vi "Initialize.vi"(7 "ChannelName":string="Setpoint.ch%d.SP", 8 "error in":errorcluster, 9 "Number of Channels":u32=1, 10 "Instance Name":string, 11 "Chiller in":refnum<class "Chiller.lvclass">) -> (0 "error out":errorcluster, 2 "Channel":T1[](array[typedef]), 3 "Chiller out":refnum<class "Chiller.lvclass">)   [LabVIEW 2023, in "Chiller.lvclass"]
uses:
  Chiller.lvclass
  Utilities/Channel.ctl
  Chiller.lvclass/Chiller.ctl
  Low Level Capabilities/OnOff/OnOff.lvclass
  Low Level Capabilities/Error/Error.lvclass
  Low Level Capabilities/Error Channels/Error Channels.lvclass
  Low Level Capabilities/Temperature/Temperature Actual Value/Temperature Actual Value.lvclass
  Low Level Capabilities/Temperature/Temperature Gradient/Temperature Gradient.lvclass
  Low Level Capabilities/Temperature/Temperature Limit/Temperature Limit.lvclass
  Low Level Capabilities/Temperature/Temperature Setpoint/Temperature Setpoint.lvclass
  Low Level Capabilities/Pressure/Pressure Actual Value/Pressure Actual Value.lvclass
  Low Level Capabilities/Pressure/Pressure Gradient/Pressure Gradient.lvclass
  Low Level Capabilities/Pressure/Pressure Limit/Pressure Limit.lvclass
  Low Level Capabilities/Pressure/Pressure Setpoint/Pressure Setpoint.lvclass
  Low Level Capabilities/Flow/Flow Actual Value/Flow Actual Value.lvclass
  Low Level Capabilities/Flow/Flow Gradient/Flow Gradient.lvclass
  Low Level Capabilities/Flow/Flow Limit/Flow Limit.lvclass
  Low Level Capabilities/Flow/Flow Setpoint/Flow Setpoint.lvclass
  Low Level Capabilities/Control Mode/Control Mode.lvclass
  Low Level Capabilities/Output Enable/Output Enable.lvclass
  Utilities/Utilities.lvlib
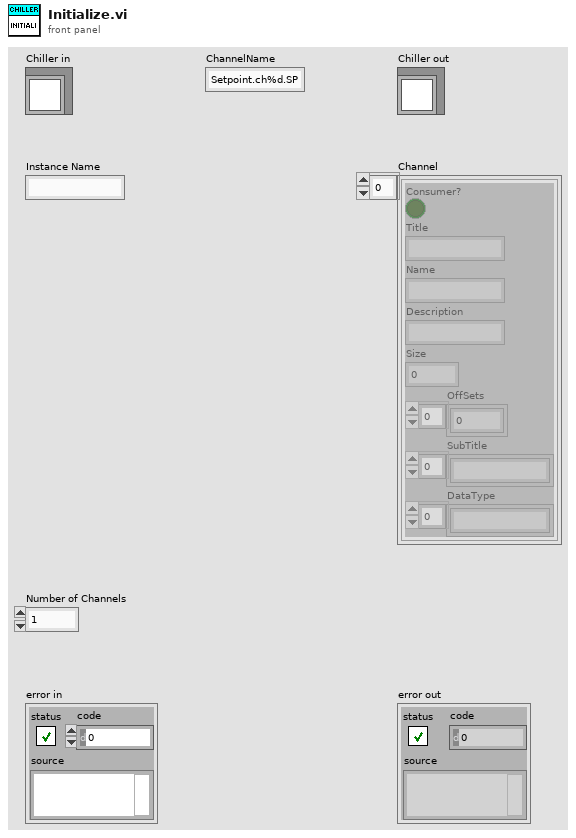
[diagram p1: front panel]
types:
  T1 = typedef "Utilities.lvlib/Channel.ctl" = cluster{"Consumer?":bool, "Title":string, "Name":string, "Description":string, "Size":i32, "OffSets":i32[], "SubTitle":string[], "DataType":string[]}
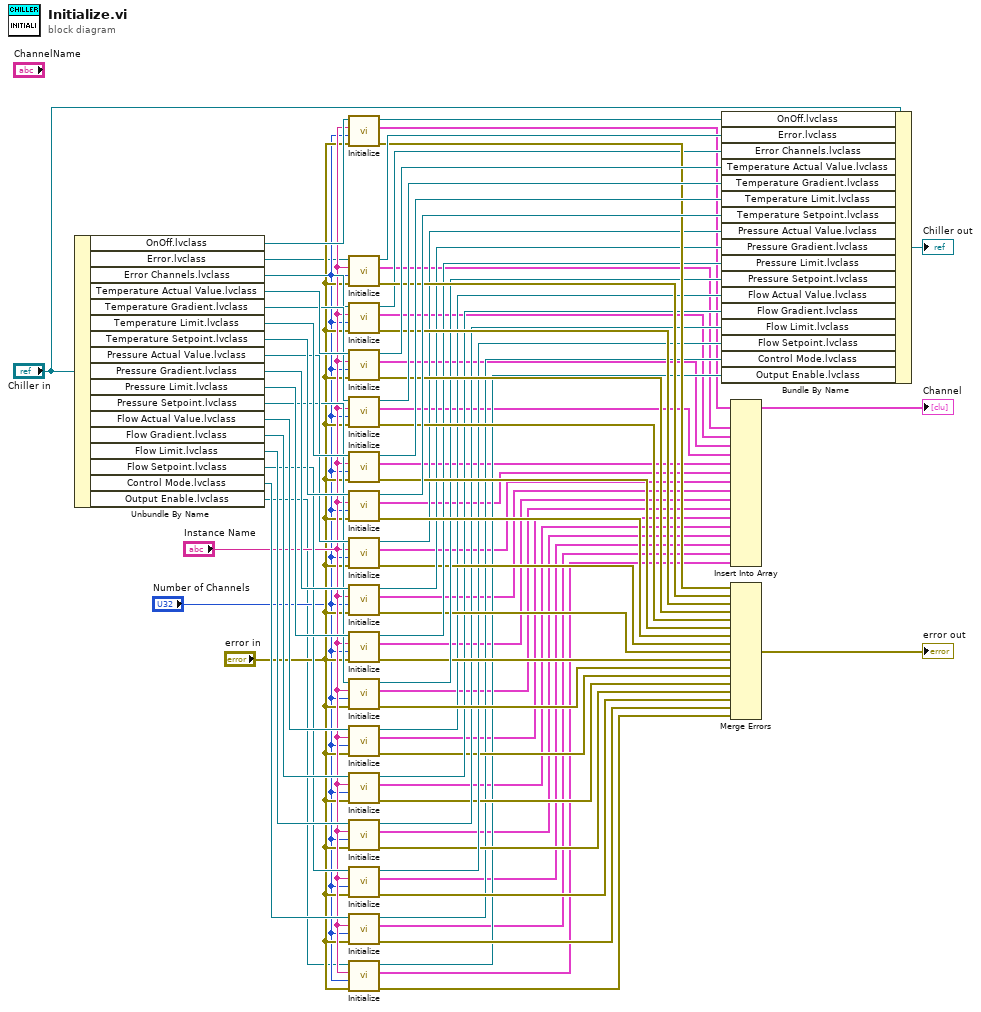
[diagram p0: block diagram]
diagram:
  n1 = Unbundle By Name("Chiller in") -> ("OnOff.lvclass"=w75:refnum<class "OnOff.lvclass">, "Error.lvclass"=w20:refnum<class "Error.lvclass">, "Error Channels.lvclass"=w58:refnum<class "Error Channels.lvclass">, "Temperature Actual Value.lvclass"=w72:refnum<class "Temperature Actual Value.lvclass">, "Temperature Gradient.lvclass"=w67:refnum<class "Temperature Gradient.lvclass">, "Temperature Limit.lvclass"=w65:refnum<class "Temperature Limit.lvclass">, "Temperature Setpoint.lvclass"=w70:refnum<class "Temperature Setpoint.lvclass">, "Pressure Actual Value.lvclass"=w55:refnum<class "Pressure Actual Value.lvclass">, "Pressure Gradient.lvclass"=w52:refnum<class "Pressure Gradient.lvclass">, "Pressure Limit.lvclass"=w50:refnum<class "Pressure Limit.lvclass">, "Pressure Setpoint.lvclass"=w48:refnum<class "Pressure Setpoint.lvclass">, "Flow Actual Value.lvclass"=w43:refnum<class "Flow Actual Value.lvclass">, "Flow Gradient.lvclass"=w42:refnum<class "Flow Gradient.lvclass">, "Flow Limit.lvclass"=w41:refnum<class "Flow Limit.lvclass">, "Flow Setpoint.lvclass"=w40:refnum<class "Flow Setpoint.lvclass">, "Control Mode.lvclass"=w29:refnum<class "Control Mode.lvclass">, "Output Enable.lvclass"=w21:refnum<class "Output Enable.lvclass">)
  n2 = call-dynamic "Initialize.vi"("error in"="error in", "Number of Channels"="Number of Channels", "Instance Name"="Instance Name", "OnOff in"=w75) -> ("error out"=w64:errorcluster, "Channel"=w18:T1[], "OnOff out"=w74:refnum<class "OnOff.lvclass">)  [unwired: 5 in]
  n3 = call-dynamic "Initialize.vi"("error in"="error in", "Number of Channels"="Number of Channels", "Instance Name"="Instance Name", "Error in"=w20) -> ("error out"=w63:errorcluster, "Channel"=w17:T1[], "Error out"=w73:refnum<class "Error.lvclass">)  [unwired: 5 in]
  n4 = call-dynamic "Initialize.vi"("error in"="error in", "Number of Channels"="Number of Channels", "Instance Name"="Instance Name", "Error Channels in"=w58) -> ("error out"=w56:errorcluster, "Channel"=w16:T1[], "Error Channels out"=w57:refnum<class "Error Channels.lvclass">)  [unwired: 5 in]
  n5 = call-dynamic "Initialize.vi"("error in"="error in", "Number of Channels"="Number of Channels", "Instance Name"="Instance Name", "Temperature Actual Value in"=w72) -> ("error out"=w62:errorcluster, "Channel"=w15:T1[], "Temperature Actual Value out"=w71:refnum<class "Temperature Actual Value.lvclass">)  [unwired: 5 in]
  n6 = call-dynamic "Initialize.vi"("error in"="error in", "Number of Channels"="Number of Channels", "Instance Name"="Instance Name", "Temperature Gradient in"=w67) -> ("error out"=w61:errorcluster, "Channel"=w14:T1[], "Temperature Gradient out"=w68:refnum<class "Temperature Gradient.lvclass">)  [unwired: 5 in]
  n7 = call-dynamic "Initialize.vi"("error in"="error in", "Number of Channels"="Number of Channels", "Instance Name"="Instance Name", "Temperature Limit in"=w65) -> ("error out"=w60:errorcluster, "Channel"=w13:T1[], "Temperature Limit out"=w66:refnum<class "Temperature Limit.lvclass">)  [unwired: 5 in]
  n8 = call-dynamic "Initialize.vi"("error in"="error in", "Number of Channels"="Number of Channels", "Instance Name"="Instance Name", "Temperature Setpoint in"=w70) -> ("error out"=w59:errorcluster, "Channel"=w12:T1[], "Temperature Setpoint out"=w69:refnum<class "Temperature Setpoint.lvclass">)  [unwired: 5 in]
  n9 = call-dynamic "Initialize.vi"("error in"="error in", "Number of Channels"="Number of Channels", "Instance Name"="Instance Name", "Pressure Actual Value in"=w55) -> ("error out"=w47:errorcluster, "Channel"=w11:T1[], "Pressure Actual Value out"=w54:refnum<class "Pressure Actual Value.lvclass">)  [unwired: 5 in]
  n10 = call-dynamic "Initialize.vi"("error in"="error in", "Number of Channels"="Number of Channels", "Instance Name"="Instance Name", "Pressure Gradient in"=w52) -> ("error out"=w46:errorcluster, "Channel"=w10:T1[], "Pressure Gradient out"=w53:refnum<class "Pressure Gradient.lvclass">)  [unwired: 5 in]
  n11 = call-dynamic "Initialize.vi"("error in"="error in", "Number of Channels"="Number of Channels", "Instance Name"="Instance Name", "Pressure Limit in"=w50) -> ("error out"=w45:errorcluster, "Channel"=w9:T1[], "Pressure Limit out"=w51:refnum<class "Pressure Limit.lvclass">)  [unwired: 5 in]
  n12 = call-dynamic "Initialize.vi"("error in"="error in", "Number of Channels"="Number of Channels", "Instance Name"="Instance Name", "Pressure Setpoint in"=w48) -> ("error out"=w44:errorcluster, "Channel"=w8:T1[], "Pressure Setpoint out"=w49:refnum<class "Pressure Setpoint.lvclass">)  [unwired: 5 in]
  n13 = call-dynamic "Initialize.vi"("error in"="error in", "Number of Channels"="Number of Channels", "Instance Name"="Instance Name", "Flow Actual Value in"=w43) -> ("error out"=w35:errorcluster, "Channel"=w7:T1[], "Flow Actual Value out"=w39:refnum<class "Flow Actual Value.lvclass">)  [unwired: 5 in]
  n14 = call-dynamic "Initialize.vi"("error in"="error in", "Number of Channels"="Number of Channels", "Instance Name"="Instance Name", "Flow Gradient in"=w42) -> ("error out"=w34:errorcluster, "Channel"=w6:T1[], "Flow Gradient out"=w38:refnum<class "Flow Gradient.lvclass">)  [unwired: 5 in]
  n15 = call-dynamic "Initialize.vi"("error in"="error in", "Number of Channels"="Number of Channels", "Instance Name"="Instance Name", "Flow Limit in"=w41) -> ("error out"=w33:errorcluster, "Channel"=w5:T1[], "Flow Limit out"=w37:refnum<class "Flow Limit.lvclass">)  [unwired: 5 in]
  n16 = call-dynamic "Initialize.vi"("error in"="error in", "Number of Channels"="Number of Channels", "Instance Name"="Instance Name", "Flow Setpoint in"=w40) -> ("error out"=w32:errorcluster, "Channel"=w4:T1[], "Flow Setpoint out"=w36:refnum<class "Flow Setpoint.lvclass">)  [unwired: 5 in]
  n17 = call-dynamic "Initialize.vi"("error in"="error in", "Number of Channels"="Number of Channels", "Instance Name"="Instance Name", "Control Mode in"=w29) -> ("error out"=w27:errorcluster, "Channel"=w3:T1[], "Control Mode out"=w28:refnum<class "Control Mode.lvclass">)  [unwired: 5 in]
  n18 = call-dynamic "Initialize.vi"("error in"="error in", "Number of Channels"="Number of Channels", "Instance Name"="Instance Name", "Output Enable in"=w21) -> ("error out"=w24:errorcluster, "Channel"=w2:T1[], "Output Enable out"=w22:refnum<class "Output Enable.lvclass">)  [unwired: 5 in]
  n19 = Bundle By Name(cluster="Chiller in", "OnOff.lvclass"=w74, "Error.lvclass"=w73, "Error Channels.lvclass"=w57, "Temperature Actual Value.lvclass"=w71, "Temperature Gradient.lvclass"=w68, "Temperature Limit.lvclass"=w66, "Temperature Setpoint.lvclass"=w69, "Pressure Actual Value.lvclass"=w54, "Pressure Gradient.lvclass"=w53, "Pressure Limit.lvclass"=w51, "Pressure Setpoint.lvclass"=w49, "Flow Actual Value.lvclass"=w39, "Flow Gradient.lvclass"=w38, "Flow Limit.lvclass"=w37, "Flow Setpoint.lvclass"=w36, "Control Mode.lvclass"=w28, "Output Enable.lvclass"=w22) -> (→"Chiller out":refnum<class "Chiller.lvclass">)
  n20 = Insert Into Array(array=w18, new element #1=w17, new element #2=w16, new element #3=w15, new element #4=w14, new element #5=w13, new element #6=w12, new element #7=w11, new element #8=w10, new element #9=w9, new element #10=w8, new element #11=w7, new element #12=w6, new element #13=w5, new element #14=w4, new element #15=w3, new element #16=w2) -> (→"Channel":T1[])  [unwired: 1 in]
  n21 = Merge Errors(w64, w63, w56, w62, w61, w60, w59, w47, w46, w45, w44, w35, w34, w33, w32, w27, w24) -> (→"error out":errorcluster)
